vi "fetch_and_translate_trigger.vi"(8 "error in (no error)":errorcluster, 11 "ExperimentControllerDL090430DAQmxTriggered in":refnum<class "ExperimentControllerDL090430DAQmxTriggered.lvclass">) -> (0 "error out":errorcluster, 1 "sender TLC type":T1=enum."ImagingMode", 2 "statechart trigger":T2, 3 "ExperimentControllerDL090430DAQmxTriggered out":refnum<class "ExperimentControllerDL090430DAQmxTriggered.lvclass">)   [LabVIEW 2010, in "ExperimentControllerDL090430DAQmxTriggered.lvclass"]
uses:
  ExperimentControllerDL090430DAQmxTriggered.lvclass
  internal_trigger_enum.ctl
  common/enumerations/top-level_component_type_enum.ctl
  GenericExperimentController/GenericExperimentController/trigger_enum.ctl
  GenericExperimentController/GenericExperimentController/GenericExperimentController.lvclass
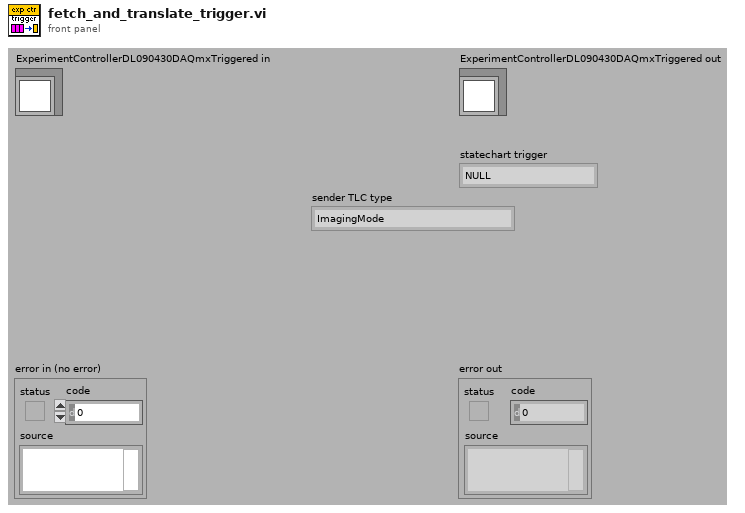
[diagram p1: front panel]
types:
  T1 = typedef "top-level_component_type_enum.ctl" = enum16{"undefined", "ImagingMode", "ScanHead", "DAQ", "ImageAssembler", "Display", "DataCollection", "Analyser", "Stimulator", "ExperimentController", "Instrument", "Stage"}
  T2 = typedef "ExperimentControllerDL090430DAQmxTriggered.lvclass/internal_trigger_enum.ctl" = enum16{"NULL", "initialise", "terminate", "proceed", "start", "stop", "start sweep", "stop sweep"}
  T3 = typedef "GenericExperimentController.lvclass/trigger_enum.ctl" = enum16{"NULL", "proceed", "prepare"}
  T4 = typedef "GenericToplevelComponent.lvclass/common_trigger_enum.ctl" = enum16{"NULL", "initialise", "terminate", "fetch command", "fetch data", "attach observer", "register as observer", "detach observer", "acknowledge", "start", "stop", "sweep started", "sweep finished", "experiment started", "experiment stopped"}
  T5 = typedef "trigger_type_enum.ctl" = enum8{"external", "internal", "common"}
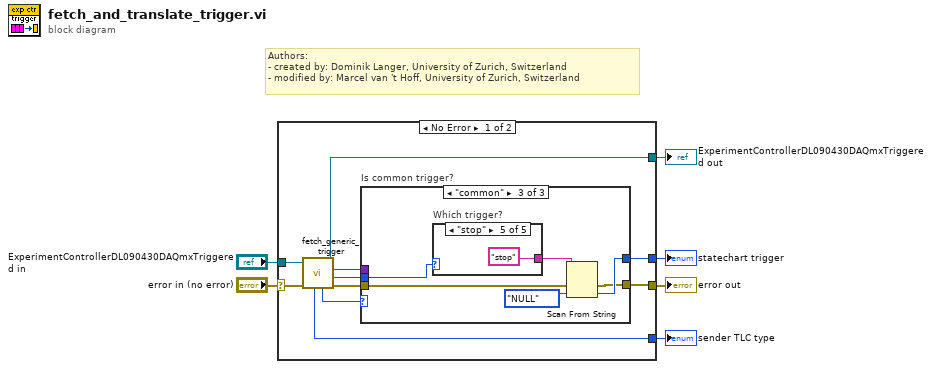
[diagram p0: block diagram]
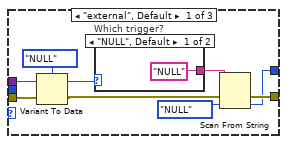
[diagram p2: hidden frame]
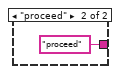
[diagram p3: hidden frame]
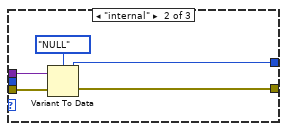
[diagram p4: hidden frame]
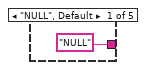
[diagram p5: hidden frame]
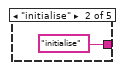
[diagram p6: hidden frame]
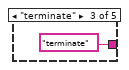
[diagram p7: hidden frame]
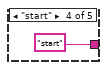
[diagram p8: hidden frame]
diagram:
  # "Authors: \n- created by: Dominik Langer, University of Zurich, Switzerland\n- modified by: Marcel van 't Hoff, University of Zurich, Switzerland"
  n1 = case shown="No Error" "error in (no error)" {
    selector: "error in (no error)" -> [w15 w45]
    tunnel: [w12 w45] -> w5
    tunnel: [w13 w44] -> w3
    tunnel: "ExperimentControllerDL090430DAQmxTriggered in" -> [w14 w44]
    tunnel: [w16 _] -> w2
    tunnel: [w7 _] -> w1
    frame No Error {
      n2 = call-dynamic "fetch_generic_trigger.vi"("error in (no error)"=w15, "GenericToplevelComponent in"=w14) -> ("error out"=w10:errorcluster, "common trigger"=w8:T4, "trigger"=w11:variant, "GenericToplevelComponent out"=w13:refnum<class "ExperimentControllerDL090430DAQmxTriggered.lvclass">, "trigger type"=w9:T5, "sender TLC type"=w7:T1)  [unwired: 3 in, 1 out]
      n3 = case "Is common trigger?" shown="\"common\"" w9 {
        tunnel: [w18 w29 w36] -> w16
        tunnel: [w19 w30 w33] -> w12
        tunnel: w11 -> [w23 w32 _]
        tunnel: w10 -> [w22 w31 w34]
        tunnel: w8 -> [_ _ w38]
        frame "external", Default {
          n4 = Variant To Data(error in=w22, Variant=w23, type=trigger_enum."NULL" ("trigger")) -> (error out=w20:errorcluster, data=w24:T3)
          n5 = case "Which trigger?" shown="\"NULL\", Default" w24 {
            tunnel: ["NULL" "proceed"] -> w21
            frame "NULL", Default {
            }
            frame "proceed" {
            }
          }
          n6 = Scan From String(input string=w21, error in=w20, default 1=internal_trigger_enum."NULL" ("statechart trigger")) -> (error out=w19:errorcluster, output 1=w18:T2)  [unwired: 2 in, 2 out]
        }
        frame "internal" {
          n7 = Variant To Data(error in=w31, Variant=w32, type=internal_trigger_enum."NULL" ("statechart trigger")) -> (error out=w30:errorcluster, data=w29:T2)
        }
        frame "common" {
          n8 = case "Which trigger?" shown="\"stop\"" w38 {
            tunnel: ["NULL" "initialise" "terminate" "start" "stop"] -> w35
            frame "NULL", Default {
            }
            frame "initialise" {
            }
            frame "terminate" {
            }
            frame "start" {
            }
            frame "stop" {
            }
          }
          n9 = Scan From String(input string=w35, error in=w34, default 1=internal_trigger_enum."NULL" ("statechart trigger")) -> (error out=w33:errorcluster, output 1=w36:T2)  [unwired: 2 in, 2 out]
        }
      }
    }
    frame Error {
    }
  }
  "error out" <- w5
  "ExperimentControllerDL090430DAQmxTriggered out" <- w3
  "statechart trigger" <- w2
  "sender TLC type" <- w1
